vi "GFITS_SetImNumFormat.vi"(8 "error in":errorcluster, 10 "imnumformat":string="%04d", 11 "Database RefNum out":T1) -> (0 "error out":errorcluster, 2 "response":string)   [LabVIEW 2016]
uses:
  DBSHAND/private/vis/DatabaseHand_RefNum.ctl
  DBSHAND/private/vis/DatabaseHand_Element_Set(string).vi
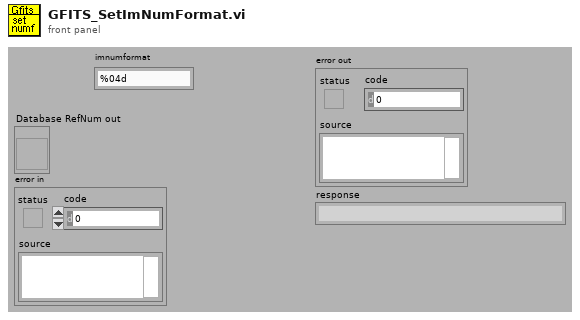
[diagram p1: front panel]
types:
  T1 = typedef "DatabaseHand_RefNum.ctl" = refnum<vi>
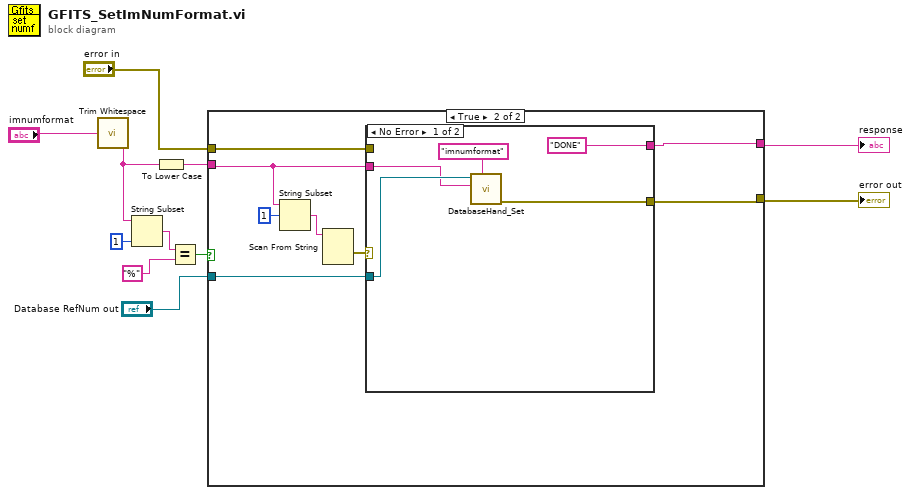
[diagram p0: block diagram]
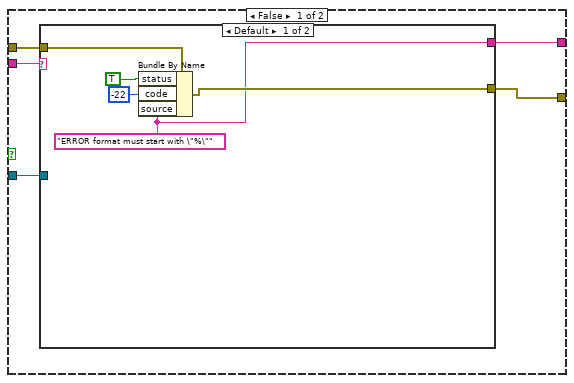
[diagram p2: hidden frame]
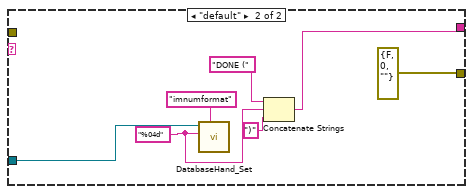
[diagram p3: hidden frame]
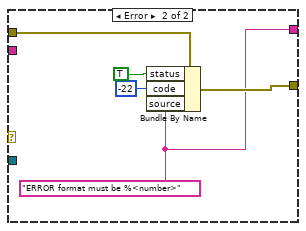
[diagram p4: hidden frame]
diagram:
  n1 = call <vilib>:"Trim Whitespace.vi"("string"="imnumformat") -> ("trimmed string"=w7:string)  [unwired: 1 in]
  n2 = String Subset(string=w7, length (rest)=1 ("length (rest)")) -> (substring=w10:string)  [unwired: 1 out]
  n3 = To Lower Case(string=w7) -> (all lower case string=w6:string)
  n4 = Equal?(x=w10, y="%") -> (x = y?=w8:bool)
  n5 = case shown="True" w8 {
    tunnel: "Database RefNum out" -> [w15 w36]
    tunnel: [w12 w35] -> w2
    tunnel: [w14 w34] -> w1
    tunnel: w6 -> [w16 w33]
    tunnel: "error in" -> [w13 w29]
    frame False {
      n6 = case shown="Default" w16 {
        tunnel: w15 -> [_ w24]
        tunnel: [w17 w23] -> w14
        tunnel: w13 -> [w19 _]
        tunnel: [w18 errorcluster {"status"=FALSE, "code"=0, "source"=""} ("error in")] -> w12
        frame Default {
          w17 = "ERROR format must start with \"%\"" ("source")
          n7 = Bundle By Name(cluster=w19, "status"=TRUE, "code"=-22, "source"=w17) -> (w18:errorcluster)
        }
        frame "default" {
          w26 = "%04d" ("value")
          n8 = call-poly "DatabaseHand_Set.vi"("name"="imnumformat", "value"=w26, "Database RefNum in"=w24) -> ()  [unwired: 5 in, 4 out]
          n9 = Concatenate Strings("DONE (" ("string"), w26, ")" ("string")) -> (w23:string)
        }
      }
    }
    frame True {
      n10 = String Subset(string=w33, offset (0)=1) -> (substring=w31:string)  [unwired: 1 out]
      n11 = Scan From String(input string=w31) -> (error out=w30:errorcluster)  [unwired: 3 in, 4 out]
      n12 = case shown="No Error" w30 {
        tunnel: w36 -> [w40 _]
        tunnel: [w39 w45] -> w35
        tunnel: ["DONE" ("filemsg") w42] -> w34
        tunnel: w33 -> [w37 _]
        tunnel: w29 -> [_ w46]
        frame No Error {
          n13 = call-poly "DatabaseHand_Set.vi"("name"="imnumformat", "value"=w37, "Database RefNum in"=w40) -> ("error out"=w39:errorcluster)  [unwired: 5 in, 3 out]
        }
        frame Error {
          w42 = "ERROR format must be %<number>" ("source")
          n14 = Bundle By Name(cluster=w46, "status"=TRUE, "code"=-22, "source"=w42) -> (w45:errorcluster)
        }
      }
    }
  }
  "error out" <- w2
  "response" <- w1
